vi "Greet World.vi"(7 "Hello (T)/Goodbye(F)":bool, 8 "error in (no error)":errorcluster, 11 "Polish in":refnum<class "Polish.lvclass">) -> (0 "error out":errorcluster, 2 "Greeting String":string, 3 "Polish out":refnum<class "Polish.lvclass">)   [LabVIEW 2019, in "Polish.lvclass"]
uses:
  Polish.lvclass
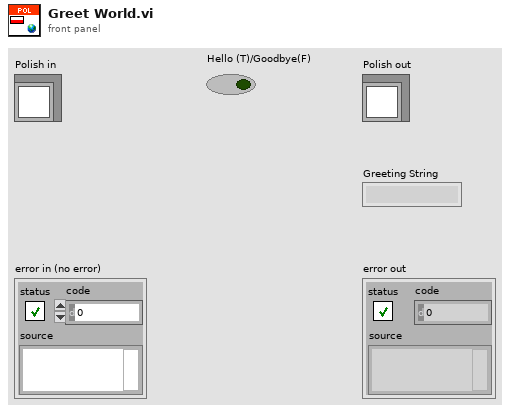
[diagram p1: front panel]
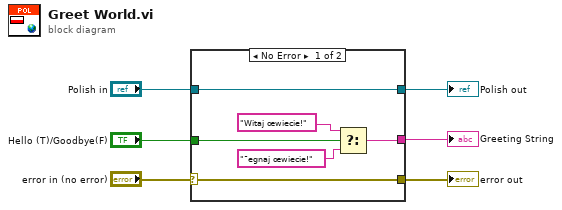
[diagram p0: block diagram]
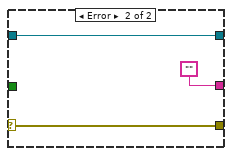
[diagram p2: hidden frame]
diagram:
  n1 = case shown="No Error" "error in (no error)" {
    selector: "error in (no error)" -> [w12 w15]
    tunnel: [w12 w15] -> w5
    tunnel: [w11 w14] -> w3
    tunnel: "Polish in" -> [w11 w14]
    tunnel: "Hello (T)/Goodbye(F)" -> [w7 _]
    tunnel: [w10 ""] -> w1
    frame No Error {
      n2 = Select(t="Witaj œwiecie!", s=w7, f="¯egnaj œwiecie!") -> (s? t:f=w10:string)
    }
    frame Error {
    }
  }
  "error out" <- w5
  "Polish out" <- w3
  "Greeting String" <- w1
